vi "Keithley 2182 Data Buffer Store and Acquire.vi"() -> ()   [LabVIEW 2021]
doc: "Stores specified measurements in buffer and reads the contents of the buffer as well as its statistics."
uses:
  <instrlib>/Keithley 2182/Keithley 2182.lvlib
panel:
  in  "milliseconds to wait":u32=1000
  in  "Selected Calculation Settings":enum32{"Linear Settings", "Percent Settings"}(tab)
  in  "Offset Value (0)":dbl
  in  "Scale Factor (1)":dbl=1.0
  in  "Units (MX)":string="MX"
  in  "Use Input Signal as Target Value (F: Disable)":bool
  in  "Target Value (1)":dbl=1.0
  in  "Selected Measurement Settings":T1(tab)
  in  "Voltage Resolution (8)":i32=8
  in  "Range Value (10)":dbl=10.0
  in  "Autorange (T: Enable)":bool=TRUE
  in  "Sensor (1: Internal)":i32(ring)=1 items=["Thermocouple", "Internal"]
  in  "Reference Junction Type (0: Internal)":i32(ring) items=["Internal", "Simulated"]
  in  "Simulated Reference Temp (23 C)":dbl=23.0
  in  "Thermocouple Type (0: J)":i32(ring) items=["J", "K", "T", "E", "R", "S", "B", "N"]
  in  "Temperature Resolution (6)":i32=6
  in  "Unit (0: Celsius)":i32(ring) items=["Celsius", "Fahrenheit", "Kelvin"]
  in  "Math Calculation (0: Linear)":i32(ring) items=["Linear", "Percent"]
  in  "Measurement (0: Voltage Channel 1)":i32(ring) items=["Voltage Channel 1", "Voltage Channel 2", "Temperature Channel 1", "Temperature Channel 2"]
  in  "Integration Rate Units (0: Line Cycles)":i32(ring) items=["Line Cycles", "Seconds"]
  in  "Integration Rate (5)":dbl=5.0
  in  "Buffer Source (0: None)":i32(ring)=1 items=["None", "Measurements", "Math Calculation"]
  out "Buffer Metadata":T2(array[cluster])
  out "Buffer":dbl[](array[numeric])
  in  "Buffer Size (10)":i32=10
  out "Mean":dbl=1.0
  out "Maximum":dbl
  out "Standard Deviation":dbl
  out "Minimum":dbl
  in  "VISA resource name":refnum<visa-resource-name>
  # "(c) 2017-2018 National Instruments.  ALL RIGHTS RESERVED."
  # "Buffer Settings"
  # "Data"
  # "Measurement Settings"
  # "Step 1: Configure Buffer\nStep 2: Configure Measurement\nStep 3: Configure Calculation (optional)\nStep 4: Adjust wait time (if necessary)\nStep 4: Read Data"
  # "Calculation Settings"
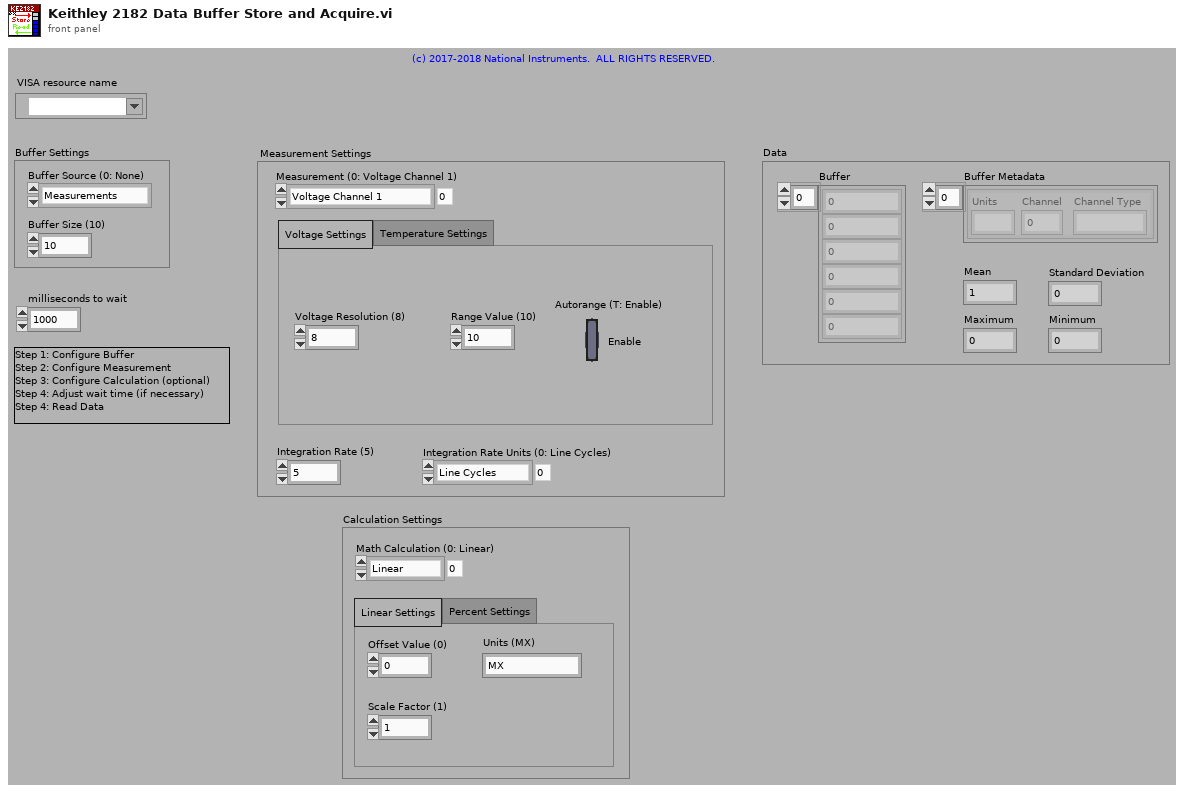
[diagram p1: front panel]
types:
  T1 = enum32{"Voltage Settings", "Temperature Settings"}
  T2 = cluster{"Units":string, "Channel":i32, "Channel Type":string}[]
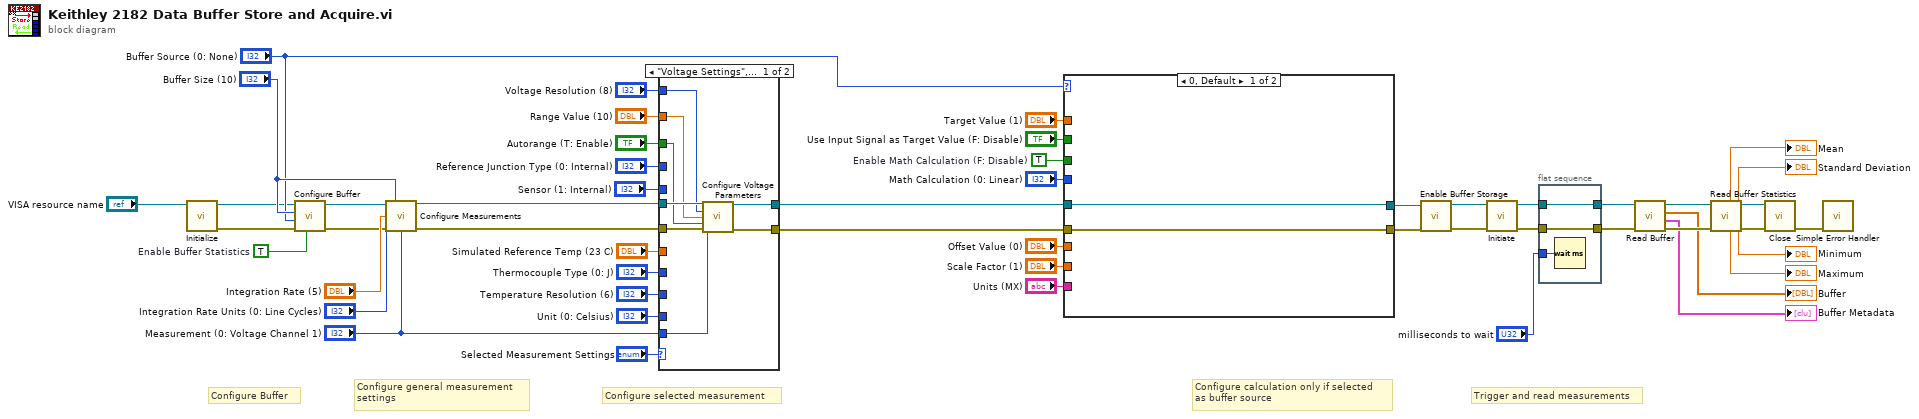
[diagram p0: block diagram]
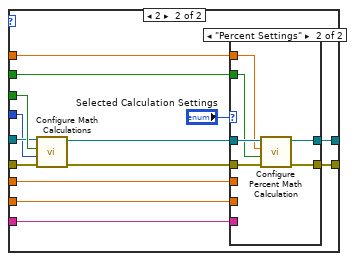
[diagram p2: hidden frame]
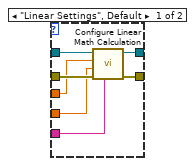
[diagram p3: hidden frame]
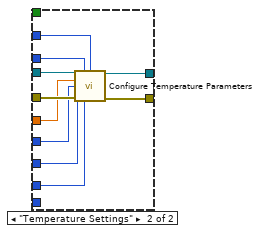
[diagram p4: hidden frame]
diagram:
  w4 = TRUE  # Enable Buffer Statistics
  w26 = TRUE  # Enable Math Calculation (F: Disable)
  # "Trigger and read measurements"
  # "Configure general measurement\nsettings"
  # "Configure Buffer"
  # "Configure calculation only if selected\nas buffer source"
  # "Configure selected measurement"
  n1 = call <instrlib>:"Initialize.vi"("VISA resource name"="VISA resource name") -> ("error out"=w17:errorcluster, "VISA resource name out"=w16:refnum<visa-resource-name>)  [unwired: 9 in]
  n2 = call <instrlib>:"Configure Buffer.vi"("Enable Buffer Statistics (0: Disable)"=w4, "error in (no error)"=w17, "Buffer Source (0: None)"="Buffer Source (0: None)", "Buffer Size (2)"="Buffer Size (10)", "VISA resource name"=w16) -> ("error out"=w41:errorcluster, "VISA resource name out"=w40:refnum<visa-resource-name>)  [unwired: 5 in]
  n3 = call <instrlib>:"Configure Measurements.vi"("VISA resource name"=w40, "Measurement (0: Voltage Channel 1)"="Measurement (0: Voltage Channel 1)", "Integration Rate (5)"="Integration Rate (5)", "Integration Rate Units (0: Line Cycles)"="Integration Rate Units (0: Line Cycles)", "error in (no error)"=w41, "Sample Count (1)"="Buffer Size (10)") -> ("VISA resource name out"=w34:refnum<visa-resource-name>, "error out"=w35:errorcluster)  [unwired: 8 in]
  n4 = case shown="\"Voltage Settings\", Default" "Selected Measurement Settings" {
    tunnel: "Voltage Resolution (8)" -> [w54 _]
    tunnel: "Range Value (10)" -> [w55 _]
    tunnel: "Autorange (T: Enable)" -> [w56 _]
    tunnel: w35 -> [w60 w70]
    tunnel: w34 -> [w59 w69]
    tunnel: [w58 w68] -> w23
    tunnel: [w57 w67] -> w24
    tunnel: "Unit (0: Celsius)" -> [_ w66]
    tunnel: "Temperature Resolution (6)" -> [_ w65]
    tunnel: "Thermocouple Type (0: J)" -> [_ w64]
    tunnel: "Simulated Reference Temp (23 C)" -> [_ w63]
    tunnel: "Sensor (1: Internal)" -> [_ w62]
    tunnel: "Reference Junction Type (0: Internal)" -> [_ w61]
    tunnel: "Measurement (0: Voltage Channel 1)" -> [w53 _]
    frame "Voltage Settings", Default {
      n5 = call <instrlib>:"Configure Voltage Parameters.vi"("VISA resource name"=w59, "Measurement (1: Voltage Channel 1)"=w53, "Voltage Resolution (8)"=w54, "Range Value (12)"=w55, "Autorange (T: Enable)"=w56, "error in (no error)"=w60) -> ("VISA resource name out"=w58:refnum<visa-resource-name>, "error out"=w57:errorcluster)  [unwired: 8 in]
    }
    frame "Temperature Settings" {
      n6 = call <instrlib>:"Configure Temperature Parameters.vi"("VISA resource name"=w69, "Sensor (0: Thermocouple)"=w62, "Reference Junction Type (0: Internal)"=w61, "Simulated Reference Temp (23 C)"=w63, "Thermocouple Type (0: J)"=w64, "Temperature Resolution (6)"=w65, "error in (no error)"=w70, "Unit (0: Celsius)"=w66) -> ("VISA resource name out"=w68:refnum<visa-resource-name>, "error out"=w67:errorcluster)  [unwired: 6 in]
    }
  }
  n7 = case shown="0, Default" "Buffer Source (0: None)" {
    tunnel: w26 -> [_ w86]
    tunnel: "Math Calculation (0: Linear)" -> [_ w83]
    tunnel: w24 -> [w72 w85]
    tunnel: w23 -> [w71 w84]
    tunnel: "Use Input Signal as Target Value (F: Disable)" -> [_ w82]
    tunnel: "Target Value (1)" -> [_ w81]
    tunnel: "Offset Value (0)" -> [_ w78]
    tunnel: "Scale Factor (1)" -> [_ w77]
    tunnel: "Units (MX)" -> [_ w76]
    tunnel: [w72 w75] -> w13
    tunnel: [w71 w74] -> w10
    frame 0, Default {
    }
    frame 2 {
      n8 = call <instrlib>:"Configure Math Calculations.vi"("error in (no error)"=w85, "Math Calculation (0: Linear)"=w83, "Enable Math Calculation (F: Disable)"=w86, "VISA resource name"=w84) -> ("error out"=w80:errorcluster, "VISA resource name out"=w79:refnum<visa-resource-name>)  [unwired: 6 in]
      n9 = case shown="\"Percent Settings\"" "Selected Calculation Settings" {
        tunnel: w82 -> [_ w95]
        tunnel: w81 -> [_ w94]
        tunnel: w80 -> [w93 w96]
        tunnel: w79 -> [w92 w97]
        tunnel: w78 -> [w91 _]
        tunnel: w77 -> [w90 _]
        tunnel: w76 -> [w89 _]
        tunnel: [w88 w99] -> w75
        tunnel: [w87 w98] -> w74
        frame "Linear Settings", Default {
          n10 = call <instrlib>:"Configure Linear Math Calculation.vi"("Units (MX)"=w89, "error in (no error)"=w93, "Offset Value (0)"=w90, "Scale Factor (1)"=w91, "VISA resource name"=w92) -> ("error out"=w88:errorcluster, "VISA resource name out"=w87:refnum<visa-resource-name>)  [unwired: 5 in]
        }
        frame "Percent Settings" {
          n11 = call <instrlib>:"Configure Percent Math Calculation.vi"("error in (no error)"=w96, "Use Input Signal as Target Value (F: Disable)"=w95, "Target Value (1)"=w94, "VISA resource name"=w97) -> ("error out"=w99:errorcluster, "VISA resource name out"=w98:refnum<visa-resource-name>)  [unwired: 6 in]
        }
      }
    }
  }
  n12 = call <instrlib>:"Enable Buffer Storage.vi"("error in (no error)"=w13, "VISA resource name"=w10) -> ("error out"=w12:errorcluster, "VISA resource name out"=w11:refnum<visa-resource-name>)  [unwired: 8 in]
  n13 = call <instrlib>:"Initiate.vi"("error in (no error)"=w12, "VISA resource name"=w11) -> ("error out"=w7:errorcluster, "VISA resource name out"=w5:refnum<visa-resource-name>)  [unwired: 8 in]
  n14 = flat-sequence {
    tunnel: "milliseconds to wait" -> [w102]
    tunnel: [w101] -> w8
    tunnel: w7 -> [w101]
    tunnel: [w100] -> w6
    tunnel: w5 -> [w100]
    frame #0 {
      n15 = Wait (ms)(milliseconds to wait=w102) -> ()  [unwired: 1 out]
    }
  }
  n16 = call <instrlib>:"Read Buffer.vi"("error in (no error)"=w8, "VISA resource name"=w6) -> ("error out"=w51:errorcluster, "Buffer Metadata"=→"Buffer Metadata":T2, "Buffer"=→"Buffer":dbl[], "VISA resource name out"=w50:refnum<visa-resource-name>)  [unwired: 6 in]
  n17 = call <instrlib>:"Read Buffer Statistics.vi"("error in (no error)"=w51, "VISA resource name"=w50) -> ("error out"=w3:errorcluster, "Minimum"=→"Minimum":dbl, "Standard Deviation"=→"Standard Deviation":dbl, "VISA resource name out"=w2:refnum<visa-resource-name>, "Maximum"=→"Maximum":dbl, "Mean"=→"Mean":dbl)  [unwired: 4 in]
  n18 = call <instrlib>:"Close.vi"("error in (no error)"=w3, "VISA resource name"=w2) -> ("error out"=w1:errorcluster)  [unwired: 9 in]
  n19 = call <vilib>:"Simple Error Handler.vi"("error in (no error)"=w1) -> ()  [unwired: 4 in, 5 out]
